vi "2283_gyro.vi"(0 "g input":dbl, 1 "g boolean":bool, 2 "angulo":dbl format="%#_13g", 3 "angulo deseado":dbl format="%#_13g") -> (5 "g output":dbl(slide) scale=-5000.0..5000.0)   [LabVIEW 2014]
uses:
  <vilib>/addons/control/pid/pid.llb/PID (DBL).vi
  <vilib>/addons/control/pid/NI_PID_pid.lvlib
panel:
  in  "PID gains":T1={"proportional gain (Kc)"=180.0, "integral time (Ti, min)"=2e-05, "derivative time (Td, min)"=3.0}
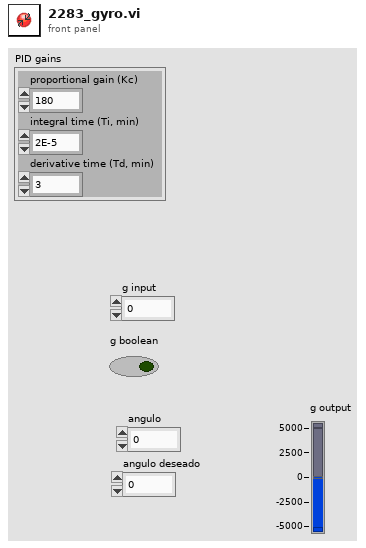
[diagram p1: front panel]
types:
  T1 = cluster{"proportional gain (Kc)":dbl, "integral time (Ti, min)":dbl, "derivative time (Td, min)":dbl}
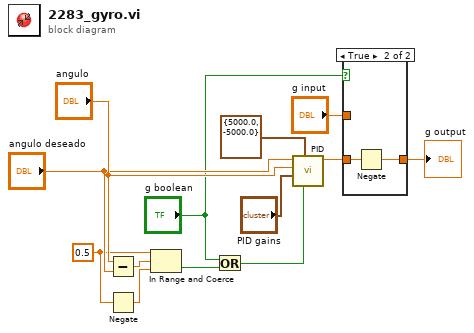
[diagram p0: block diagram]
diagram:
  w4 = 0.5
  n1 = Subtract(x="angulo", y="angulo deseado") -> (x-y=w8:dbl)
  n2 = Negate(x=w4) -> (-x=w5:dbl)
  n3 = In Range and Coerce(upper limit=w4, x=w8, lower limit=w5) -> (In Range?=w2:bool)  [unwired: 1 out]
  n4 = Or(x="g boolean", y=w2) -> (x .or. y?=w3:bool)
  n5 = call-poly <vilib>:"PID.vi"("reinitialize? (F)"=w3, "output range"=cluster{"output high":dbl, "output low":dbl} {"output high"=5000.0, "output low"=-5000.0}, "PID gains"="PID gains", "process variable"="angulo", "setpoint"="angulo deseado") -> ("output"=w10:dbl)  [unwired: 5 in, 1 out]
  n6 = case shown="True" "g boolean" {
    tunnel: [w14 w15] -> w12
    tunnel: w10 -> [_ w16]
    tunnel: "g input" -> [w14 _]
    frame False {
    }
    frame True {
      n7 = Negate(x=w16) -> (-x=w15:dbl)
    }
  }
  "g output" <- w12
